vi "EventDrivenStateMachine.vi"() -> ()   [LabVIEW 2014]
uses:
  My Typedefs/StateTypeDef.ctl
panel:
  in  "Stop Application":bool
  in  "Pause State Machine":bool
  in  "Play State Machine":bool
  out "State":T1=enum."Init"
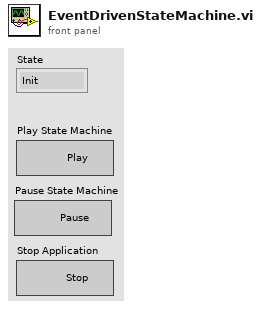
[diagram p1: front panel]
types:
  T1 = typedef "StateTypeDef.ctl" = enum16{"Idle", "Stop", "Play", "Init"}
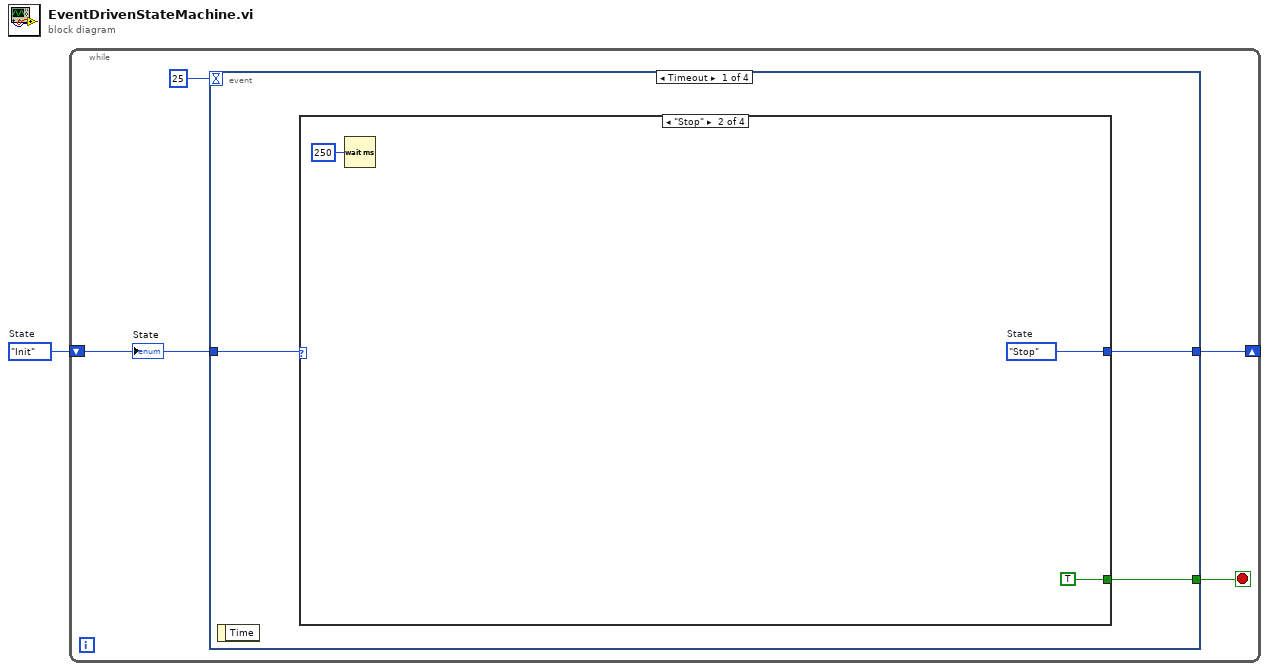
[diagram p0: block diagram]
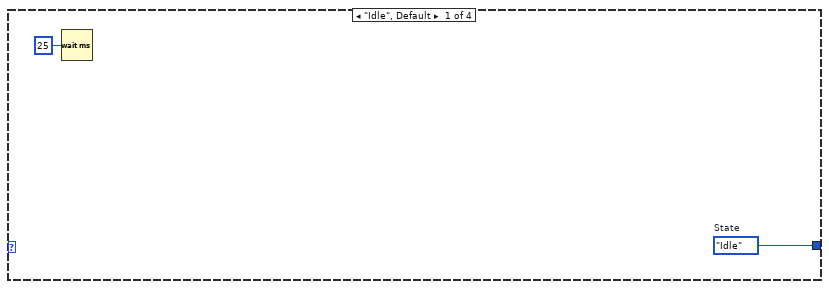
[diagram p2: hidden frame]
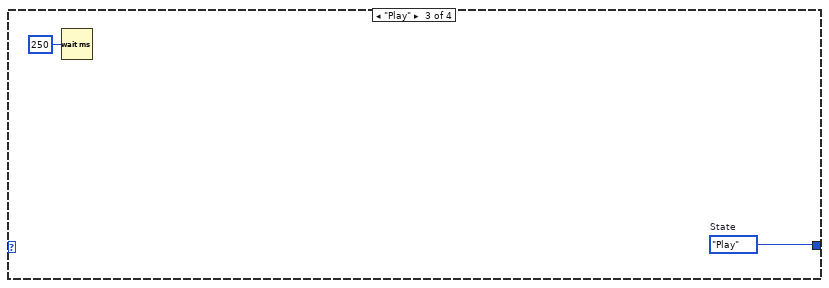
[diagram p3: hidden frame]
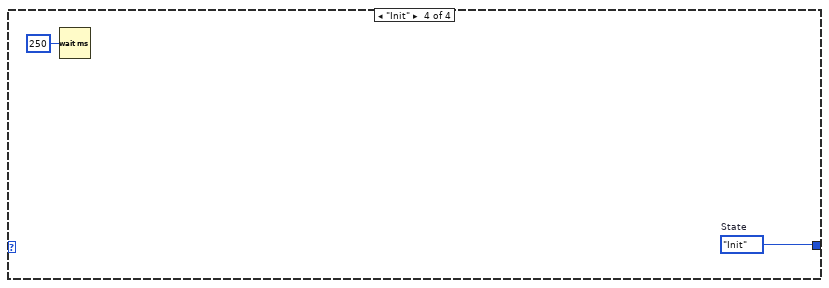
[diagram p4: hidden frame]
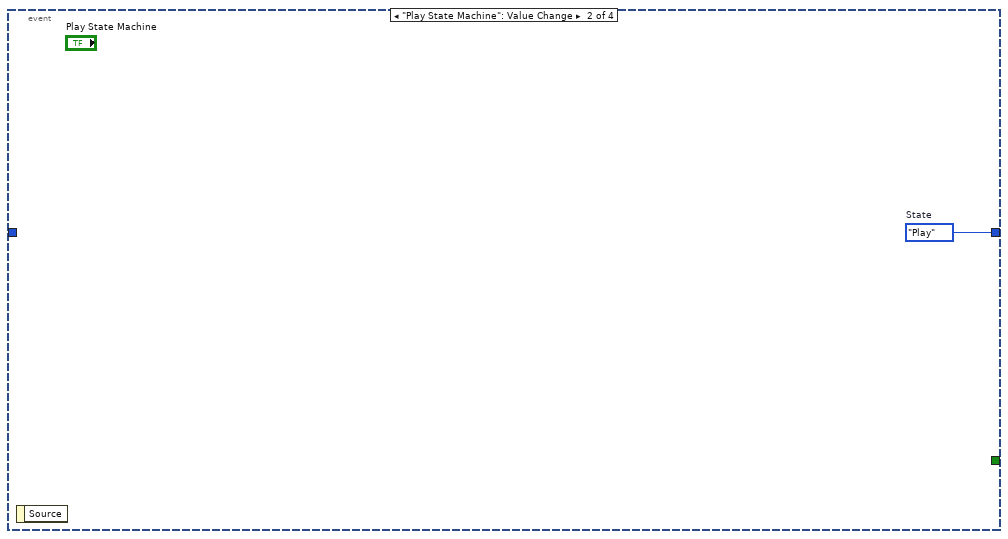
[diagram p5: hidden frame]
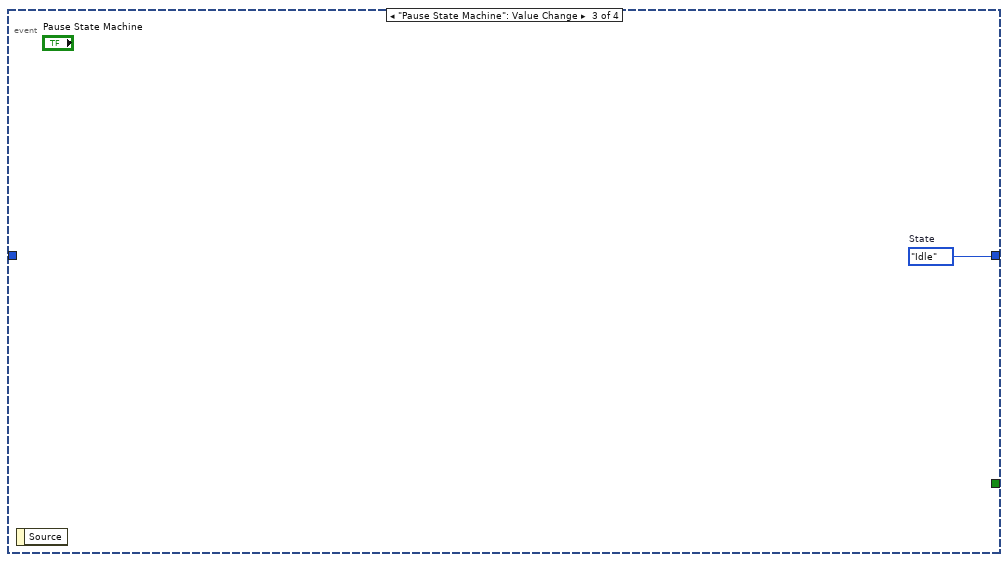
[diagram p6: hidden frame]
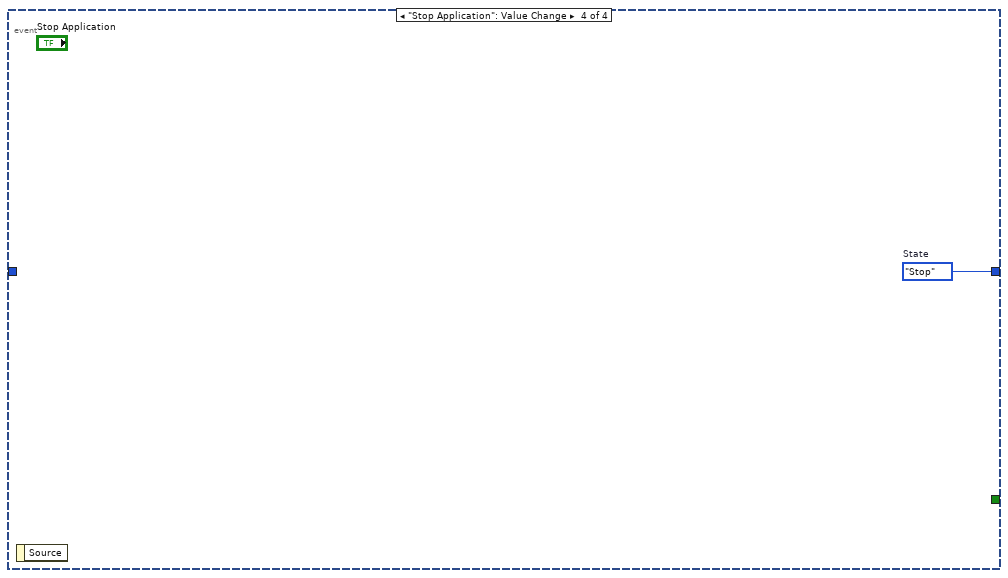
[diagram p7: hidden frame]
diagram:
  w1 = StateTypeDef."Init"  # State
  n1 = while {
    shift-right: [w3] -> _
    shift-left: w1 -> [w4]
    stop <- w2 stop-if-true
    n2 = event shown="[0] Timeout" {
      selector: _ -> [_ _ _ _]
      dyn-events: _ -> [_ _ _ _]
      timeout: 25 -> [_ _ _ _]
      tunnel: w4 -> [w8 _ _ _]
      tunnel: [w7 w18 w19 w20] -> w3
      tunnel: [w6 _ _ _] -> w2
      event Timeout {
        n3 = event-data() -> ()  [unwired: 1 in, 1 out]
        n4 = case shown="\"Stop\"" w8 {
          tunnel: [w10 w13 w15 w17] -> w7
          tunnel: [_ TRUE _ _] -> w6
          frame "Idle", Default {
            w10 = StateTypeDef."Idle"  # State
            n5 = Wait (ms)(milliseconds to wait=u32 25) -> ()  [unwired: 1 out]
          }
          frame "Stop" {
            w13 = StateTypeDef."Stop"  # State
            n6 = Wait (ms)(milliseconds to wait=u32 250) -> ()  [unwired: 1 out]
          }
          frame "Play" {
            w15 = StateTypeDef."Play"  # State
            n7 = Wait (ms)(milliseconds to wait=u32 250) -> ()  [unwired: 1 out]
          }
          frame "Init" {
            w17 = StateTypeDef."Init"  # State
            n8 = Wait (ms)(milliseconds to wait=u32 250) -> ()  [unwired: 1 out]
          }
        }
      }
      event "Play State Machine": Value Change {
        w18 = StateTypeDef."Play"  # State
        n9 = event-data() -> ()  [unwired: 1 in, 1 out]
      }
      event "Pause State Machine": Value Change {
        w19 = StateTypeDef."Idle"  # State
        n10 = event-data() -> ()  [unwired: 1 in, 1 out]
      }
      event "Stop Application": Value Change {
        w20 = StateTypeDef."Stop"  # State
        n11 = event-data() -> ()  [unwired: 1 in, 1 out]
      }
    }
    "State" <- w4
  }
